vi "WriteInSharedVarBOOL.vi"(8 "entrée d'erreur (pas d'erreur)":errorcluster, 9 "données en entrée":bool, 11 "refnum de variable partagée en entrée":refnum<k21>) -> (0 "sortie d'erreur":errorcluster)   [LabVIEW 2013]
doc: "Ce VI permet d'ouvrir une variable partagée, d'y écrire un booléen, et de la fermer. VI créé pour Open ModBus Eth 2.20 avec lesquel plusieurs variables partagées par le serveur OPC ne peuvent être ouvertes simultanément (ce qui était le cas avec la version 2.14)\nAV 18/11/2013"
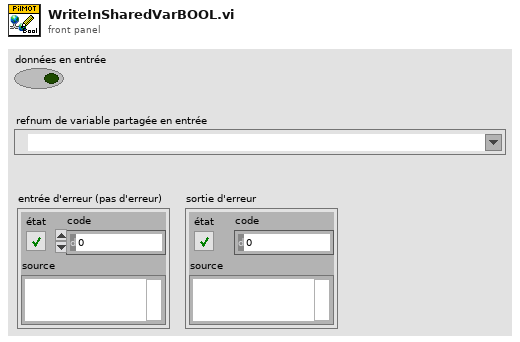
[diagram p1: front panel]
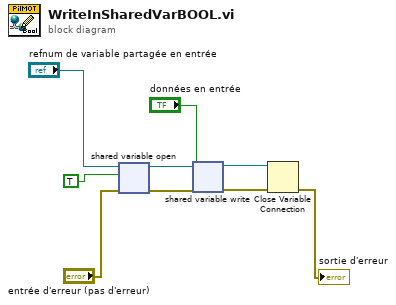
[diagram p0: block diagram]
diagram:
  n1 = shared-variable-open("refnum de variable partagée en entrée", "entrée d'erreur (pas d'erreur)", TRUE) -> (w3:refnum<k21>, w5:errorcluster)  [unwired: 1 in]
  n2 = shared-variable-write(w3, w5, "données en entrée") -> (w2:refnum<k21>, w4:errorcluster)
  n3 = Close Variable Connection(8:w4, 11:w2) -> (0:→"sortie d'erreur":errorcluster)
